vi "Read T_Out.vi"(8 "error in (no error)":errorcluster, 11 "CIFFIFO in":refnum<class "CIFfifo.lvclass">) -> (0 "error out":errorcluster, 2 "T_Out":u64, 3 "CIFFIFO out":refnum<class "CIFfifo.lvclass">)   [LabVIEW 2021, in "CIFfifo.lvclass"]
uses:
  CIFfifo.lvclass
  CIFfifo.lvclass/CIFfifo.ctl
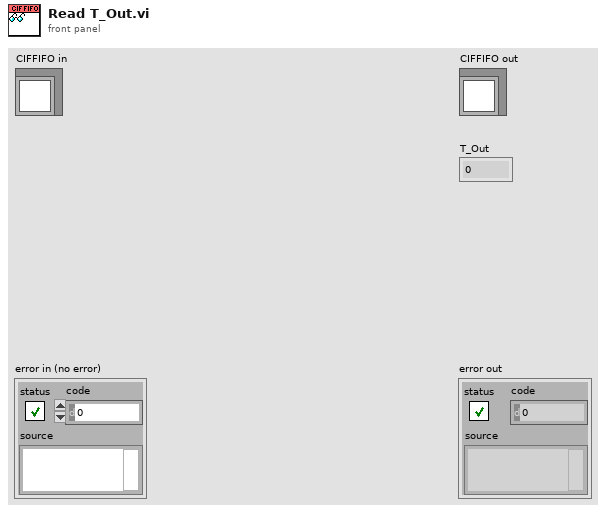
[diagram p1: front panel]
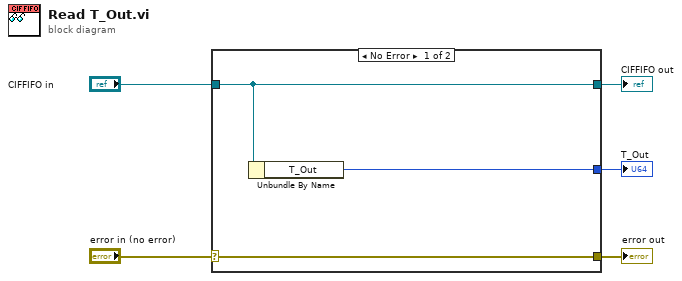
[diagram p0: block diagram]
diagram:
  n1 = case shown="No Error" "error in (no error)" {
    selector: "error in (no error)" -> [w8 w9]
    tunnel: [w8 w9] -> w4
    tunnel: [w7 w10] -> w2
    tunnel: "CIFFIFO in" -> [w7 w10]
    tunnel: [w6 _] -> w1
    frame No Error {
      n2 = Unbundle By Name(w7) -> ("T_Out"=w6:u64)
    }
    frame Error {
    }
  }
  "error out" <- w4
  "CIFFIFO out" <- w2
  "T_Out" <- w1
